vi "DefenderArea.vi"(6 "Number of Defenders\nWithout Duelist":i32, 8 "error in (no error)":errorcluster, 9 "RobotRef":refnum<class "Robot.lvclass">, 10 "Game in":refnum<class "Game.lvclass">, 11 "DefenderAreaRole in":refnum<class "DefenderAreaRole.lvclass">) -> (0 "error out":errorcluster, 2 "Robot out":refnum<class "Robot.lvclass">, 3 "DefenderAreaRole out":refnum<class "DefenderAreaRole.lvclass">)   [LabVIEW 2024, in "DefenderAreaRole.lvclass"]
uses:
  DefenderAreaRole.lvclass
  C:/Users/ROBOIME2/Documents/SSL ROBOIME/SSL_AI/Role_class/Role.lvclass
  Robot_class/Robot.lvclass
  Game_class/Game.lvclass
  Role_class/Role.lvclass/Role.ctl
  DefendAreaTactic_class/Read States.vi
  Role_class/Read Tacticbook.vi
  Role_class/Read tactic_index.vi
  Role_class/Write Tacticbook.vi
  Role_class/Write tactic_index.vi
  Tacticbook_class/Tacticbook.lvclass
  DefendAreaTactic_class/DefendAreaTactic.lvclass
panel:
  out "Game out":refnum<class "Game.lvclass">
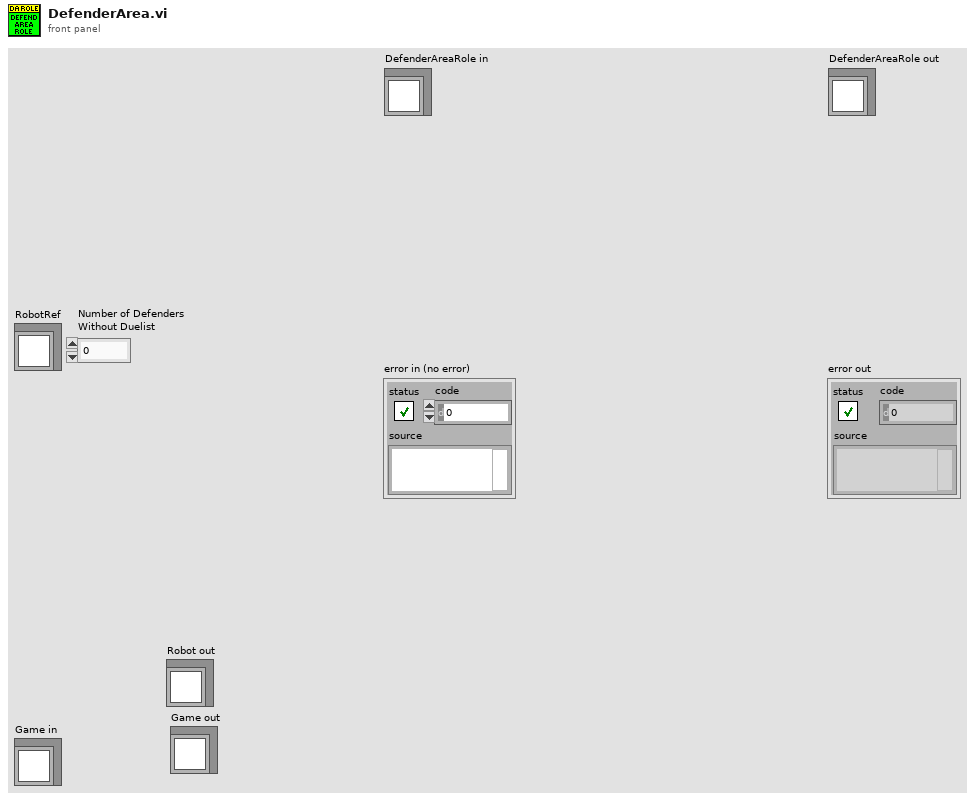
[diagram p1: front panel]
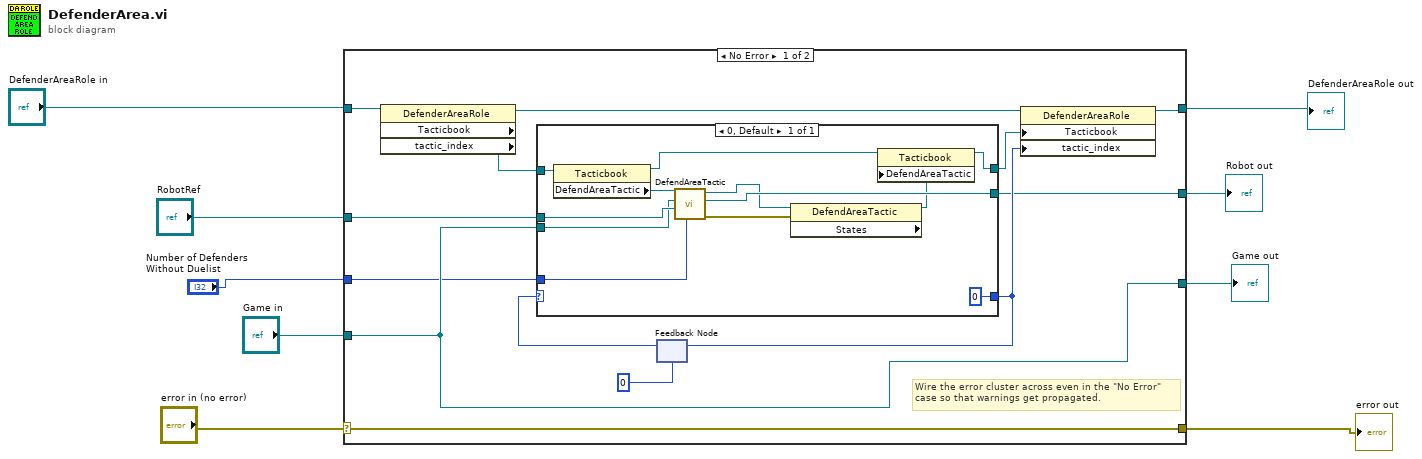
[diagram p0: block diagram]
diagram:
  n1 = case shown="No Error" "error in (no error)" {
    selector: "error in (no error)" -> [w22 w38]
    tunnel: [w22 w38] -> w3
    tunnel: [w20 w37] -> w6
    tunnel: "DefenderAreaRole in" -> [w21 w37]
    tunnel: "RobotRef" -> [w14 w36]
    tunnel: [w13 w36] -> w9
    tunnel: [w11 w35] -> w8
    tunnel: "Game in" -> [w11 w35]
    tunnel: "Number of Defenders\nWithout Duelist" -> [w10 _]
    frame No Error {
      # "Wire the error cluster across even in the \"No Error\"\ncase so that warnings get propagated."
      n2 = property class="DefenderAreaRole" props=["Tacticbook", "tactic_index"](reference=w21) -> (reference out=w19:refnum<class "DefenderAreaRole.lvclass">, "Tacticbook"=w16:refnum<class "Tacticbook.lvclass">)  [unwired: 1 in, 2 out]
      n3 = feedback #1(0) -> (w17:i32)
      n4 = case shown="0, Default" w17 {
        tunnel: [0] -> w15
        tunnel: w16 -> [w34]
        tunnel: w14 -> [w32]
        tunnel: [w31] -> w13
        tunnel: [w26] -> w12
        tunnel: w11 -> [w25]
        tunnel: w10 -> [w23]
        frame 0, Default {
          n5 = property class="Tacticbook"(reference=w34) -> (reference out=w28:refnum<class "Tacticbook.lvclass">, "DefendAreaTactic"=w33:refnum<class "DefendAreaTactic.lvclass">)  [unwired: 1 in, 1 out]
          n6 = call "DefendAreaTactic.vi"("Number of Defenders\nWithout Duelist"=w23, "Robot"=w32, "Game in"=w25, "DefendAreaTactic in"=w33) -> ("error out"=w30:errorcluster, "Robot out"=w31:refnum<class "Robot.lvclass">, "DefendAreaTactic out"=w29:refnum<class "DefendAreaTactic.lvclass">)  [unwired: 5 in]
          n7 = property class="DefendAreaTactic" props=["States"](reference=w29, error in=w30) -> (reference out=w27:refnum<class "DefendAreaTactic.lvclass">)  [unwired: 2 out]
          n8 = property class="Tacticbook"(reference=w28, "DefendAreaTactic"=w27) -> (reference out=w26:refnum<class "Tacticbook.lvclass">)  [unwired: 1 in, 1 out]
        }
      }
      n9 = feedback-in #1(w15) -> ()
      n10 = property class="DefenderAreaRole"(reference=w19, "Tacticbook"=w12, "tactic_index"=w15) -> (reference out=w20:refnum<class "DefenderAreaRole.lvclass">)  [unwired: 1 in, 1 out]
    }
    frame Error {
    }
  }
  "error out" <- w3
  "DefenderAreaRole out" <- w6
  "Robot out" <- w9
  "Game out" <- w8
